vi "move axe.vi"(9 "Axe":dbl, 10 "Vitesse":dbl, 11 "Angle":dbl) -> ()   [LabVIEW 2015]
uses:
  Variable globale.vi
  <userlib>/ICNC/ICNC2.lvlib
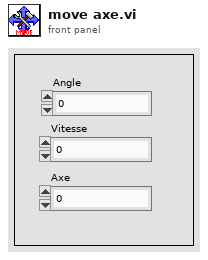
[diagram p1: front panel]
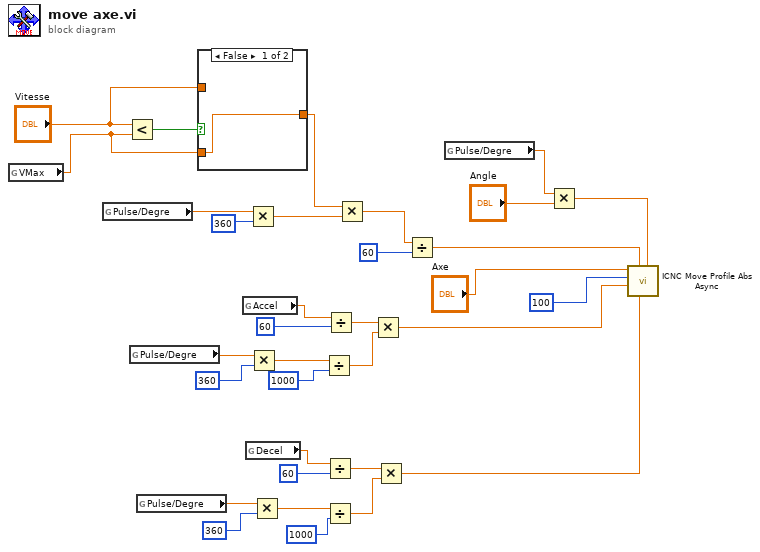
[diagram p0: block diagram]
diagram:
  n1 = global read "Variable globale.vi" "VMax"() -> (w12:dbl)
  n2 = global read "Variable globale.vi" "Pulse/Degre"() -> (w22:dbl)
  n3 = Less?(x="Vitesse", y=w12) -> (x < y?=w14:bool)
  n4 = global read "Variable globale.vi" "Pulse/Degre"() -> (w31:dbl)
  n5 = global read "Variable globale.vi" "Pulse/Degre"() -> (w25:dbl)
  n6 = case shown="False" w14 {
    tunnel: "Vitesse" -> [_ w35]
    tunnel: w12 -> [w34 _]
    tunnel: [w34 w35] -> w8
    frame False {
    }
    frame True {
    }
  }
  n7 = global read "Variable globale.vi" "Accel"() -> (w20:dbl)
  n8 = global read "Variable globale.vi" "Decel"() -> (w7:dbl)
  n9 = Multiply(x=w22, y=360) -> (x*y=w9:dbl)
  n10 = Multiply(x=w31, y=360) -> (x*y=w11:dbl)
  n11 = Multiply(x=w25, y=360) -> (x*y=w10:dbl)
  n12 = Divide(x=w11, y=1000) -> (x/y=w32:dbl)
  n13 = Divide(x=w7, y=60) -> (x/y=w27:dbl)
  n14 = Divide(x=w10, y=1000) -> (x/y=w26:dbl)
  n15 = Divide(x=w20, y=60) -> (x/y=w18:dbl)
  n16 = Multiply(x=w8, y=w9) -> (x*y=w17:dbl)
  n17 = Multiply(x=w18, y=w32) -> (x*y=w3:dbl)
  n18 = Multiply(x=w27, y=w26) -> (x*y=w2:dbl)
  n19 = Divide(x=w17, y=60) -> (x/y=w5:dbl)
  n20 = global read "Variable globale.vi" "Pulse/Degre"() -> (w16:dbl)
  n21 = Multiply(x=w16, y="Angle") -> (x*y=w6:dbl)
  n22 = call <userlib>:"ICNC Move Profile Abs Async.vi"("Position"=w6, "Decel"=w2, "Speed"=w5, "Accel"=w3, "FStartStop"=100, "Axe"="Axe") -> ()  [unwired: 4 in, 2 out]
